vi "释放队列.vi"(0 "error in (no error)":errorcluster caption="错误输入（无错误）", 3 "控制盒（队列） 输入":refnum<class "控制盒（队列）.lvclass"> caption="DNL_LabVIEW Object in") -> (7 "error out":errorcluster caption="错误输出", 10 "控制盒（队列） 输出":refnum<class "控制盒（队列）.lvclass"> caption="DNL_LabVIEW Object out")   [LabVIEW 2011, in "控制盒（队列）.lvclass"]
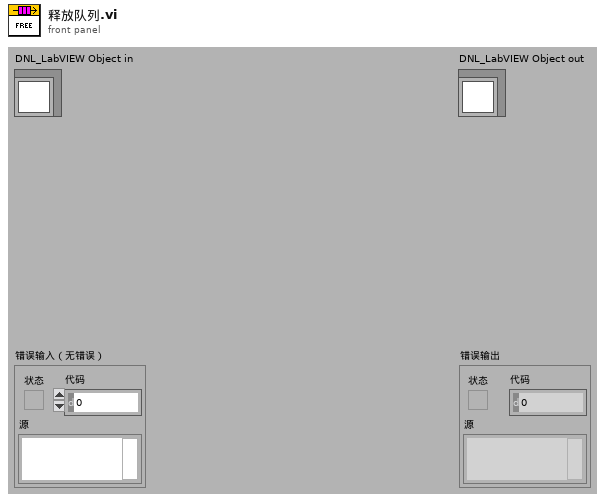
[diagram p1: front panel]
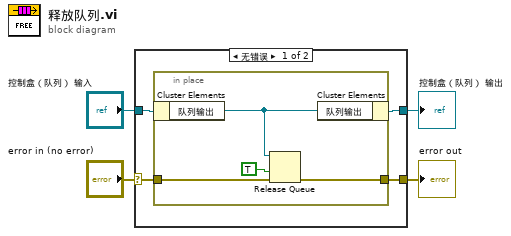
[diagram p0: block diagram]
diagram:
  n1 = case shown="无错误" "error in (no error)" {
    selector: "error in (no error)" -> [w7 w14]
    tunnel: [w6 w14] -> w3
    tunnel: [w5 w13] -> w1
    tunnel: "控制盒（队列） 输入" -> [w8 w13]
    frame No Error {
      n2 = in-place {
        in-place-border: w7 -> [w12]
        in-place-border: [w11] -> w6
        n3 = in-place-cluster #1(w8) -> ("队列输出"=w9:refnum<queue>)
        n4 = Release Queue(queue=w9, force destroy? (F)=TRUE ("强制销毁？(F)"), error in (no error)=w12) -> (error out=w11:errorcluster)  [unwired: 2 out]
        n5 = in-place-cluster #1("队列输出"=w9) -> (w5:refnum<class "控制盒（队列）.lvclass">)
      }
    }
    frame Error {
    }
  }
  "error out" <- w3
  "控制盒（队列） 输出" <- w1
